vi "SRV_SRV_Loops Notifier.vi"(6 "Notifier Methods":T1, 8 "error in (no error)":errorcluster, 9 "Cancelled? (F)":bool) -> (0 "error out":errorcluster, 1 "Cancelled?":bool)   [LabVIEW 2014]
doc: "Manges the \"SRV_Loops\" notifier used for some of the synchronization between the two loops.\n\n\nAuthor: Mike Schultz - Logic PD"
uses:
  SRV_SRV_Loops Notifier Methods.ctl
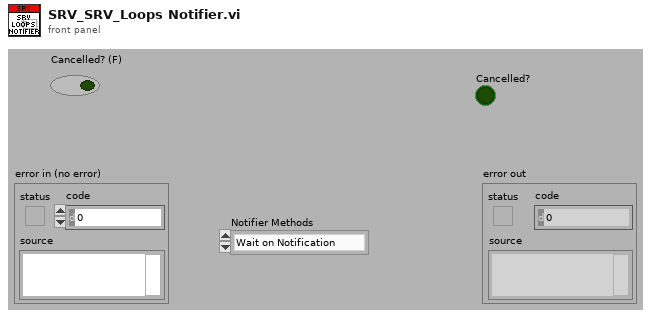
[diagram p1: front panel]
types:
  T1 = typedef "SRV_SRV_Loops Notifier Methods.ctl" = enum16{"Wait on Notification", "Send Notification", "Release Notifier"}
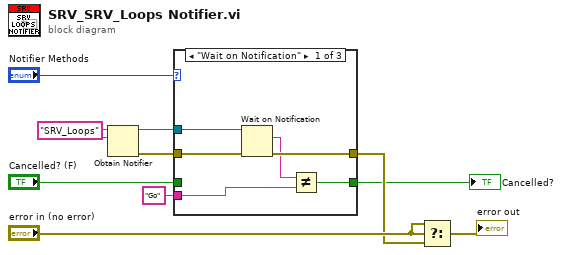
[diagram p0: block diagram]
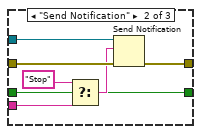
[diagram p2: hidden frame]
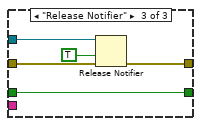
[diagram p3: hidden frame]
diagram:
  w10 = "SRV_Loops" ("name (unnamed)")
  n1 = Obtain Notifier(name (unnamed)=w10, notification data type=w10) -> (notifier out=w6:refnum<notifier>, error out=w5:errorcluster)  [unwired: 2 in, 1 out]
  n2 = case shown="\"Wait on Notification\"" "Notifier Methods" {
    tunnel: [w15 w23 w28] -> w7
    tunnel: w6 -> [w14 w22 w26]
    tunnel: w5 -> [w16 w21 w27]
    tunnel: "Cancelled? (F)" -> [_ w17 w24]
    tunnel: "Go" ("notification") -> [w12 w18 _]
    tunnel: [w11 w17 w24] -> w1
    frame "Wait on Notification" {
      n3 = Wait on Notification(notifier=w14, error in (no error)=w16) -> (notification=w13:string, error out=w15:errorcluster)  [unwired: 2 in, 2 out]
      n4 = Not Equal?(x=w13, y=w12) -> (x != y?=w11:bool)
    }
    frame "Send Notification" {
      n5 = Select(t="Stop" ("notification"), s=w17, f=w18) -> (s? t:f=w20:string)
      n6 = Send Notification(notification=w20, notifier=w22, error in (no error)=w21) -> (error out=w23:errorcluster)  [unwired: 1 out]
    }
    frame "Release Notifier" {
      n7 = Release Notifier(notifier=w26, force destroy? (F)=TRUE, error in (no error)=w27) -> (error out=w28:errorcluster)  [unwired: 2 out]
    }
  }
  "Cancelled?" <- w1
  n8 = Select(t="error in (no error)", s="error in (no error)", f=w7) -> (s? t:f=→"error out":errorcluster)
